vi "createLoopArrayIOL.vi"(0 "Bgstart":dbl, 1 "Step Increase pos":dbl, 2 "Increase pos":dbl, 3 "Bgstop":dbl, 5 "nbpoint1":dbl, 7 "Bgstop2":dbl, 9 "Sweeps":i32=1, 11 "Nb loops":i32, 12 "Step Increase neg":dbl, 13 "Increase neg":dbl, 14 "nbpoint2":dbl) -> (8 "Outarray":dbl[](array[numeric]))   [LabVIEW 2011]
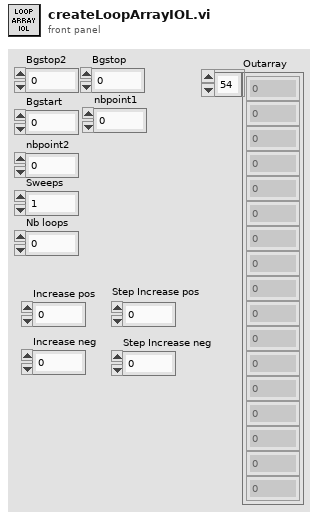
[diagram p1: front panel]
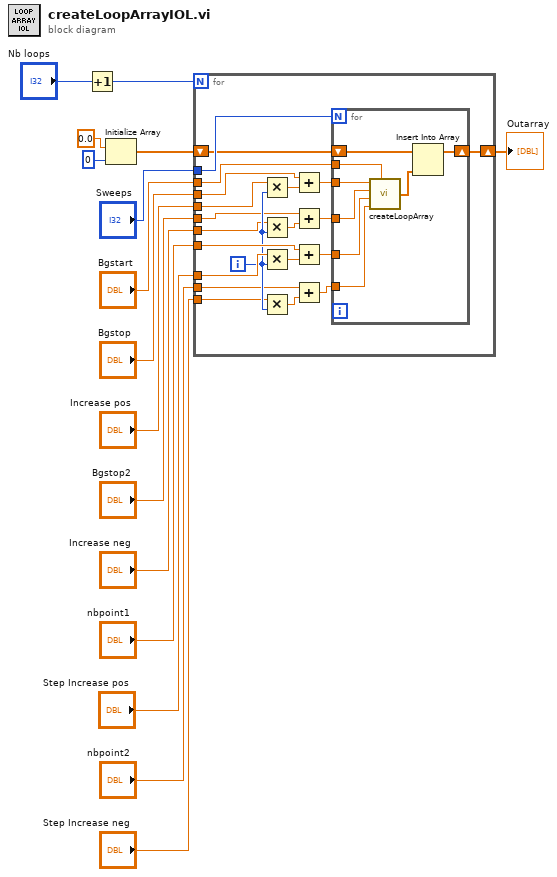
[diagram p0: block diagram]
diagram:
  n1 = Increment(x="Nb loops") -> (x+1=w1:i32)
  n2 = Initialize Array(0.0 ("element"), 0 ("index")) -> (w3:dbl[])
  n3 = for {
    N: w1 -> [_]
    tunnel: "Sweeps" -> [w37]
    tunnel: "Bgstop" -> [w34]
    tunnel: "Increase pos" -> [w36]
    tunnel: "Step Increase pos" -> [w32]
    tunnel: "nbpoint1" -> [w30]
    tunnel: "Bgstart" -> [w28]
    tunnel: "Increase neg" -> [w26]
    tunnel: "Step Increase neg" -> [w25]
    tunnel: "nbpoint2" -> [w22]
    tunnel: "Bgstop2" -> [w21]
    shift-right: [w17] -> w2
    shift-left: w3 -> [w18]
    i -> [w27]
    n4 = Multiply(x=w36, y=w27) -> (x*y=w35:dbl)
    n5 = Multiply(x=w26, y=w27) -> (x*y=w23:dbl)
    n6 = Multiply(x=w32, y=w27) -> (x*y=w31:dbl)
    n7 = Multiply(x=w25, y=w27) -> (x*y=w24:dbl)
    n8 = Add(x=w34, y=w35) -> (x+y=w33:dbl)
    n9 = Add(x=w21, y=w23) -> (x+y=w20:dbl)
    n10 = Add(x=w30, y=w31) -> (x+y=w29:dbl)
    n11 = Add(x=w22, y=w24) -> (x+y=w19:dbl)
    n12 = for {
      N: w37 -> [_]
      shift-right: [w38] -> w17
      shift-left: w18 -> [w39]
      tunnel: w33 -> [w43]
      tunnel: w29 -> [w45]
      tunnel: w28 -> [w44]
      tunnel: w20 -> [w42]
      tunnel: w19 -> [w41]
      n13 = call "createLoopArray.vi"("Bgstop"=w43, "Bgstop2"=w42, "nbpoint1"=w45, "nbpoint2"=w41, "Bgstart"=w44) -> ("Outarray"=w40:dbl[])
      n14 = Insert Into Array(array=w39, new element=w40) -> (w38:dbl[])  [unwired: 1 in]
    }
  }
  "Outarray" <- w2
